vi "Save-Recall Instrument Setup.vi"(8 "error in (no error)":errorcluster, 9 "Memory Location (0: Position 0)":u16(ring) items=["0", "1", "2", "3", "4", "5", "6", "7", "8", "9", "10", "11", "12", "13", "14", "15"], 10 "Operation (0 : Save)":u16(ring) items=["Save", "Recall"], 11 "VISA resource name":refnum<visa-resource-name>) -> (0 "error out":errorcluster, 3 "VISA resource name out":refnum<visa-resource-name>)   [LabVIEW 2020, in "Agilent 681x Series.lvlib"]
doc: "Saves instrument settings to or recalls instrument settings from the selected memory location."
uses:
  <instrlib>/Agilent 681x Series/Agilent 681x Series.lvlib
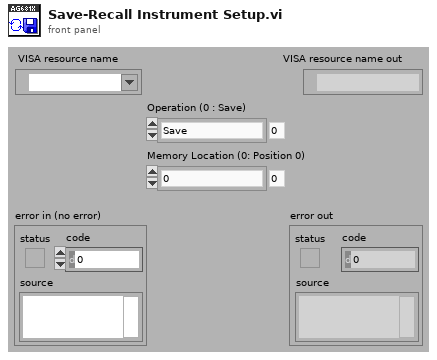
[diagram p1: front panel]
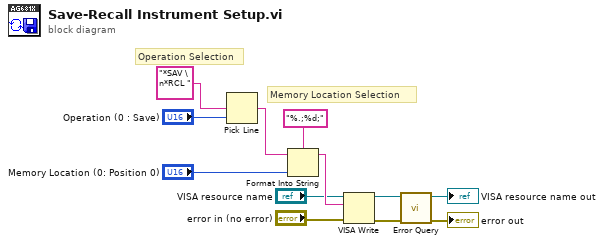
[diagram p0: block diagram]
diagram:
  # "Memory Location Selection"
  # "Operation Selection"
  n1 = Pick Line(multi-line string="*SAV \n*RCL ", line index="Operation (0 : Save)") -> (output string=w7:string)  [unwired: 1 in]
  n2 = Format Into String(format string="%.;%d;", initial string=w7, "Memory Location (0: Position 0)") -> (resulting string=w8:string)  [unwired: 1 in, 1 out]
  n3 = VISA Write(VISA resource name="VISA resource name", write buffer=w8, error in (no error)="error in (no error)") -> (VISA resource name out=w4:refnum<visa-resource-name>, error out=w5:errorcluster)  [unwired: 1 out]
  n4 = call <instrlib>:"Error Query.vi"("error in (no error)"=w5, "VISA resource name"=w4) -> ("error out"=→"error out":errorcluster, "VISA resource name out"=→"VISA resource name out":refnum<visa-resource-name>)  [unwired: 6 in, 2 out]
